vi "volumeDown.vi"(8 "error in (no error)":errorcluster, 11 "BasicRemote in":refnum<class "BasicRemote.lvclass">) -> (0 "error out":errorcluster, 3 "BasicRemote out":refnum<class "BasicRemote.lvclass">)   [LabVIEW 2018, in "BasicRemote.lvclass"]
uses:
  BasicRemote.lvclass
  BasicRemote.lvclass/BasicRemote.ctl
  Device Class/Device.lvclass
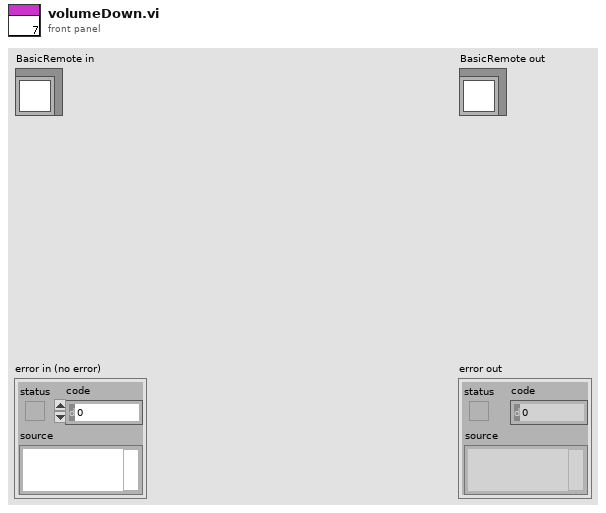
[diagram p1: front panel]
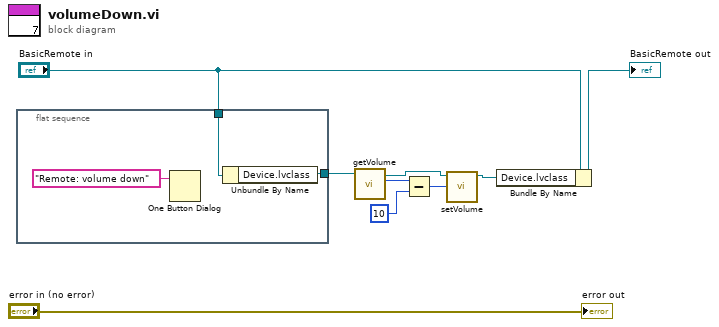
[diagram p0: block diagram]
diagram:
  n1 = flat-sequence {
    tunnel: "BasicRemote in" -> [w11]
    tunnel: [w10] -> w7
    frame #0 {
      n2 = One Button Dialog(message="Remote: volume down") -> ()  [unwired: 1 in, 1 out]
      n3 = Unbundle By Name(w11) -> ("Device.lvclass"=w10:refnum<class "Device.lvclass">)
    }
  }
  n4 = call-dynamic "getVolume.vi"("Device in"=w7) -> ("volume"=w6:i32, "Device out"=w3:refnum<class "Device.lvclass">)  [unwired: 8 in, 1 out]
  n5 = Subtract(x=w6, y=10) -> (x-y=w4:i32)
  n6 = call-dynamic "setVolume.vi"("volume"=w4, "Device in"=w3) -> ("Device out"=w1:refnum<class "Device.lvclass">)  [unwired: 8 in, 1 out]
  n7 = Bundle By Name(cluster="BasicRemote in", "Device.lvclass"=w1) -> (→"BasicRemote out":refnum<class "BasicRemote.lvclass">)
  "error out" <- "error in (no error)"
